vi "Set Font.vi"(7 "Sheet Name":string, 8 "error in":errorcluster, 9 "Font":T1={"Bold"=enum."default", "Italic"=enum."default", "Underline"=enum."default", "Color"=0, "Size"=-1.0, "Name"=""}, 10 "Cell Address":string, 11 "SpreadsheetDoc in":refnum<k24>) -> (0 "error out":errorcluster, 3 "SpreadsheetDoc out":refnum<k24>)   [LabVIEW 2021, in "Open Xml.lvlib"]
uses:
  Source/Open Xml.lvlib
  D:/git/Open-Xml-LabVIEW/dll/DocumentFormat.OpenXml.dll
  dll/DocumentFormat.OpenXml.dll
  Source/Font.ctl
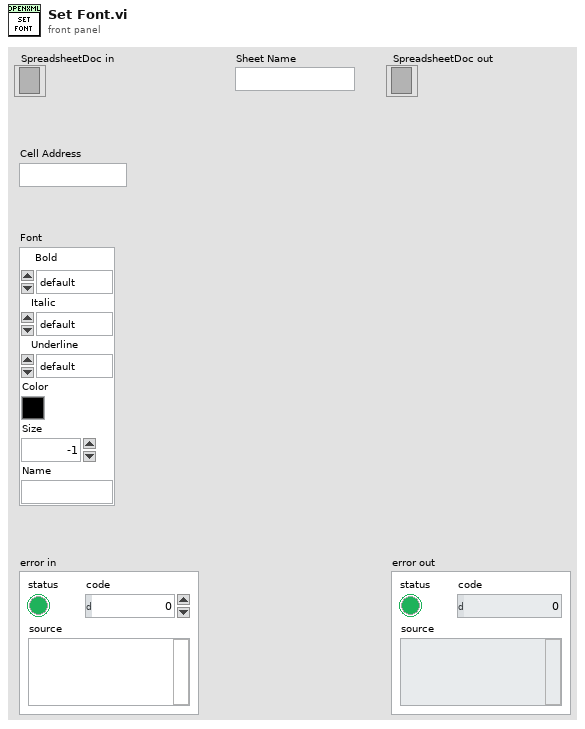
[diagram p1: front panel]
types:
  T1 = typedef "Open Xml.lvlib/Font.ctl" = cluster{"Bold":enum16{"bold", "regular", "default"}, "Italic":enum16{"italic", "regular", "default"}, "Underline":enum16{"single", "double", "singleAccounting", "doubleAccounting", "none", "default"}, "Color":u32, "Size":dbl, "Name":string}
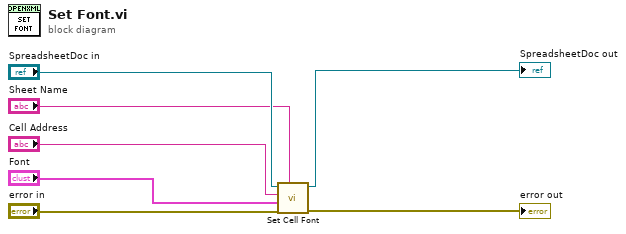
[diagram p0: block diagram]
diagram:
  n1 = call "Set Cell Font.vi"("Sheet Name"="Sheet Name", "error in"="error in", "Font"="Font", "Cell Address"="Cell Address", "SpreadsheetDoc in"="SpreadsheetDoc in") -> ("error out"=→"error out":errorcluster, "SpreadsheetDoc out"=→"SpreadsheetDoc out":refnum<k24>)  [unwired: 5 in]
